vi "Assert In Range.vi"(7 "Message (\"\")":string, 8 "error in (no error)":errorcluster, 9 "Minimum":ext, 10 "Actual":ext, 11 "Maximum":ext) -> (0 "error out":errorcluster)   [LabVIEW 2017, in "Transparent Assertions.lvlib" / "Assertions.lvlib"]
doc: "Asserts that a value is greater than or equal to the maximum value and less than or equal to the minimum value. Returns an error if the assertion fails, and optionally appends a custom message to the error."
uses:
  Assertions.lvlib
  Constraints/Logical And/Logical And.lvclass
  C:/Users/pasca/Projects/Home/TransparentAssertions/src/Transparent Assertions/Constraints/Binary Operator/Binary Operator.lvclass
  Constraints/Logical Or/Logical Or.lvclass
  C:/Users/pasca/Projects/Home/TransparentAssertions/src/Transparent Assertions/Constraints/Constraint/Constraint.lvclass
  Constraints/Is Less Than/Is Less Than.lvclass
  Constraints/IsEqual/IsEqual.lvclass
  Constraints/Is Greater Than/Is Greater Than.lvclass
  Constraints/Binary Operator/Binary Operator.lvclass
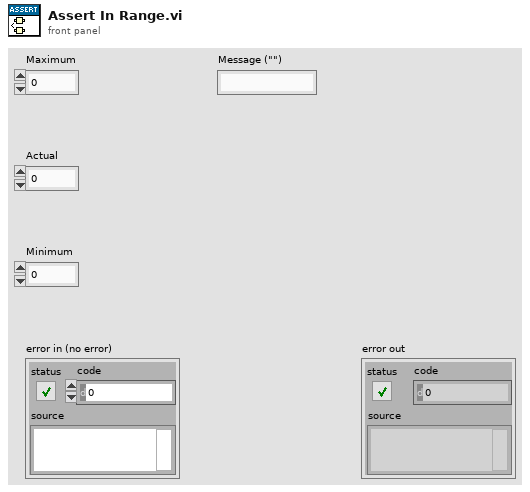
[diagram p1: front panel]
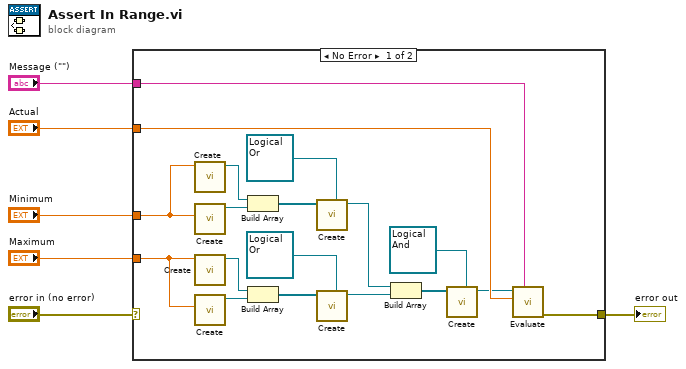
[diagram p0: block diagram]
diagram:
  n1 = case shown="No Error" "error in (no error)" {
    selector: "error in (no error)" -> [_ w25]
    tunnel: "Actual" -> [w24 _]
    tunnel: [w23 w25] -> w6
    tunnel: "Message (\"\")" -> [w22 _]
    tunnel: "Minimum" -> [w21 _]
    tunnel: "Maximum" -> [w20 _]
    frame No Error {
      n2 = call "Create.vi"("Expected"=w21) -> ("Is Greater Than"=w17:refnum<class "Is Greater Than.lvclass">)  [unwired: 9 in, 1 out]
      n3 = call "Create.vi"("Expected"=w21) -> ("IsEqual"=w16:refnum<class "IsEqual.lvclass">)  [unwired: 9 in, 1 out]
      n4 = call "Create.vi"("Expected"=w20) -> ("Is Less Than"=w19:refnum<class "Is Less Than.lvclass">)  [unwired: 9 in, 1 out]
      n5 = call "Create.vi"("Expected"=w20) -> ("IsEqual"=w18:refnum<class "IsEqual.lvclass">)  [unwired: 9 in, 1 out]
      n6 = Build Array(w17, w16) -> (w14:refnum<class "Constraint.lvclass">[])
      n7 = Build Array(w19, w18) -> (w15:refnum<class "Constraint.lvclass">[])
      n8 = call "Create.vi"("Binary Operator in"=refnum<class "Logical Or.lvclass"> refnum ("Transparent Assertions.lvlib:Constraints.lvlib:Logical Or.lvclass"), "Constraints"=w14) -> ("Binary Operator"=w11:refnum<class "Logical Or.lvclass">)  [unwired: 8 in, 1 out]
      n9 = call "Create.vi"("Binary Operator in"=refnum<class "Logical Or.lvclass"> refnum ("Transparent Assertions.lvlib:Constraints.lvlib:Logical Or.lvclass"), "Constraints"=w15) -> ("Binary Operator"=w12:refnum<class "Logical Or.lvclass">)  [unwired: 8 in, 1 out]
      n10 = Build Array(w11, w12) -> (w10:refnum<class "Logical Or.lvclass">[])
      n11 = call "Create.vi"("Binary Operator in"=refnum<class "Logical And.lvclass"> refnum ("Transparent Assertions.lvlib:Constraints.lvlib:Logical And.lvclass"), "Constraints"=w10) -> ("Binary Operator"=w9:refnum<class "Logical And.lvclass">)  [unwired: 8 in, 1 out]
      n12 = call-dynamic "Evaluate.vi"("Message (\"\")"=w22, "Actual"=w24, "Constraint in"=w9) -> ("error out"=w23:errorcluster)  [unwired: 7 in, 1 out]
    }
    frame Error {
    }
  }
  "error out" <- w6
